vi "Get Cell (Boolean).vi"(6 "Column":i32, 8 "error in (no error)":errorcluster, 9 "Row":i32, 10 "Sheet Reference":refnum<k24>) -> (0 "error out":errorcluster, 2 "Sheet Reference out":refnum<k24>, 5 "Value":bool)   [LabVIEW 2014]
uses:
  C:/Users/LENOVO/Desktop/CodeSpace GUI/LVExcel/Resources/net40/NPOI.dll
  Resources/net40/NPOI.dll
  <vilib>/ErrorRing/Error Ring.xnode
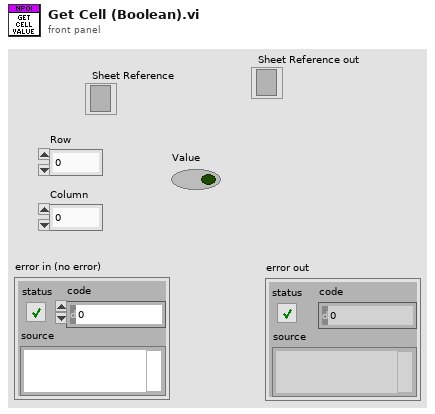
[diagram p1: front panel]
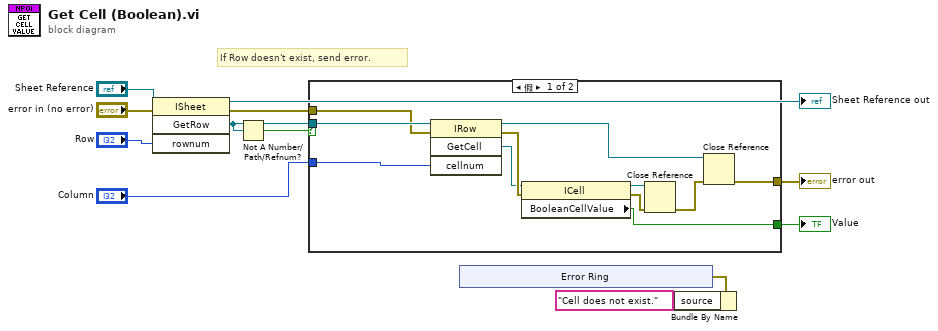
[diagram p0: block diagram]
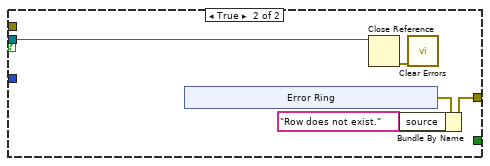
[diagram p2: hidden frame]
diagram:
  # "If Row doesn't exist, send error."
  n1 = invoke class="ISheet" method="GetRow"(reference="Sheet Reference", error in="error in (no error)", "rownum"="Row") -> (reference out=→"Sheet Reference out":refnum<k24>, error out=w5:errorcluster, "GetRow"=w10:refnum<k24>)  [unwired: 1 in, 1 out]
  n2 = Not A Number/Path/Refnum?(number/path/refnum=w10) -> (NaN/Path/Refnum?=w4:bool)
  n3 = case shown="假" w4 {
    tunnel: "Column" -> [w22 _]
    tunnel: [w20 w25] -> w11
    tunnel: w10 -> [w19 w28]
    tunnel: w5 -> [w18 _]
    tunnel: [w13 _] -> w1
    frame False {
      n4 = invoke class="IRow" method="GetCell"(reference=w19, error in=w18, "cellnum"=w22) -> (reference out=w23:refnum<k24>, error out=w17:errorcluster, "GetCell"=w16:refnum<k24>)  [unwired: 1 in, 1 out]
      n5 = property class="ICell"(reference=w16, error in=w17) -> (reference out=w14:refnum<k24>, error out=w15:errorcluster, "BooleanCellValue"=w13:bool)
      n6 = Close Reference(reference=w14, error in (no error)=w15) -> (error out=w21:errorcluster)
      n7 = Close Reference(reference=w23, error in (no error)=w21) -> (error out=w20:errorcluster)
    }
    frame True {
      n8 = xnode "Error Ring"() -> ("错误输出"=w26:errorcluster)
      n9 = Close Reference(reference=w28) -> (error out=w27:errorcluster)  [unwired: 1 in]
      n10 = Bundle By Name(cluster=w26, "source"="Row does not exist.") -> (w25:errorcluster)
      n11 = call <vilib>:"Clear Errors.vi"("error in (no error)"=w27) -> ()  [unwired: 5 in, 2 out]
    }
  }
  "error out" <- w11
  "Value" <- w1
  n12 = xnode "Error Ring"() -> ("错误输出"=w2:errorcluster)
  n13 = Bundle By Name(cluster=w2, "source"="Cell does not exist.") -> ()  [unwired: 1 out]
